vi "LogError.vi"(8 "error in (no error)":errorcluster, 11 "TCP_Server in":refnum<class "TCP_Server.lvclass">) -> (0 "error out":errorcluster, 3 "TCP_Server out":refnum<class "TCP_Server.lvclass">)   [LabVIEW 2023, in "TCP_Server.lvlib" / "TCP_Server.lvclass"]
uses:
  TCP_Server.lvclass
  TCP_Server.lvclass/TCP_Server.ctl
  SimpleErrorLogger/SimpleErrorLogger Messages/LogError Msg/LogError Msg.lvclass
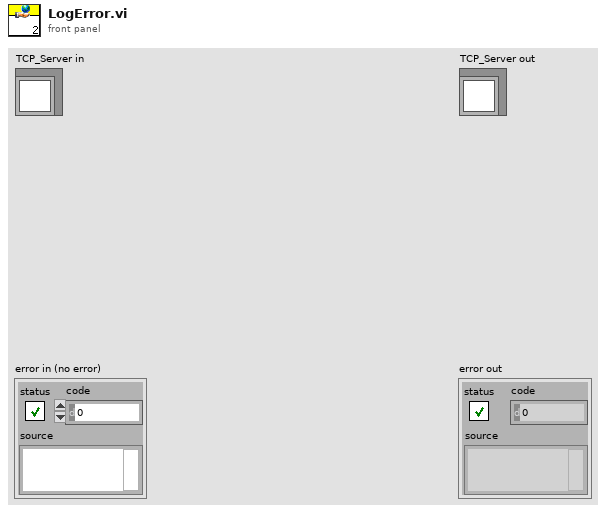
[diagram p1: front panel]
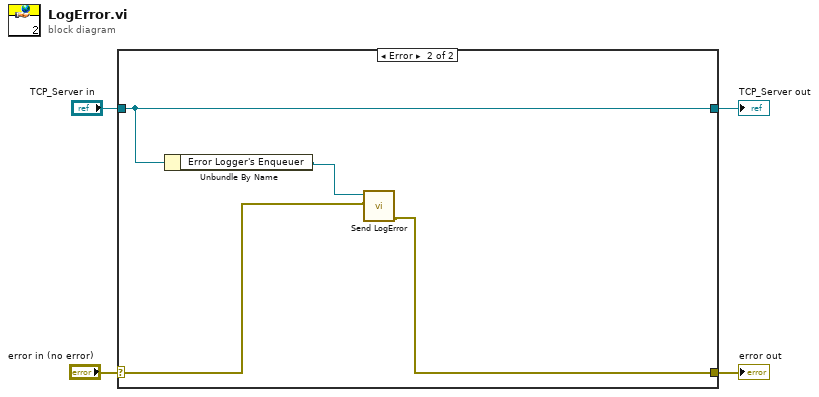
[diagram p0: block diagram]
diagram:
  n1 = case shown="Error" "error in (no error)" {
    selector: "error in (no error)" -> [w6 w8]
    tunnel: [w6 w7] -> w3
    tunnel: [w5 w9] -> w1
    tunnel: "TCP_Server in" -> [w5 w9]
    frame No Error {
    }
    frame Error {
      n2 = Unbundle By Name(w9) -> ("Error Logger's Enqueuer"=w10:refnum<class "Message Enqueuer.lvclass">)
      n3 = call "Send LogError.vi"("error"=w8, "Message Enqueuer"=w10) -> ("error out"=w7:errorcluster)  [unwired: 8 in, 1 out]
    }
  }
  "error out" <- w3
  "TCP_Server out" <- w1
